vi "new encoder test harness.vi"(5 "input2":bool=TRUE, 6 "Tick Count(Ticks)":u32, 7 "input1":bool=TRUE, 8 "ticks":u32[](array[numeric])=[0, 0], 9 "switch encoders (F)":bool, 10 "rising edge (T)":bool=TRUE, 11 "history in":bool[](array[boolean])=[FALSE, FALSE, FALSE, FALSE, FALSE, FALSE, FALSE, FALSE, FALSE, FALSE, FALSE, FALSE, FALSE, FALSE, FALSE, FALSE, FALSE, FALSE, FALSE, FALSE, FALSE, FALSE, FALSE, FALSE, FALSE, FALSE, FALSE, FALSE, FALSE, FALSE, FALSE, FALSE, FALSE, FALSE, FALSE, FALSE, FALSE, FALSE, FALSE, FALSE, FALSE, FALSE, FALSE, FALSE, FALSE, FALSE, FALSE, FALSE, FALSE, FALSE, FALSE, FALSE, FALSE, FALSE, FALSE, FALSE, FALSE, FALSE, FALSE, FALSE, FALSE, FALSE, FALSE, FALSE, FALSE, FALSE, FALSE, FALSE, FALSE, FALSE, FALSE, FALSE, FALSE, FALSE, FALSE, FALSE, FALSE, FALSE, FALSE, FALSE, FALSE, FALSE, FALSE, FALSE, FALSE, FALSE, FALSE, FALSE, FALSE, FALSE, FALSE, FALSE, FALSE, FALSE, FALSE, FALSE, FALSE, FALSE, FALSE, FALSE]) -> (0 "ticks out":u32[](array[numeric]), 2 "edge detected":bool, 3 "history out":bool[](array[boolean]))   [LabVIEW 2018]
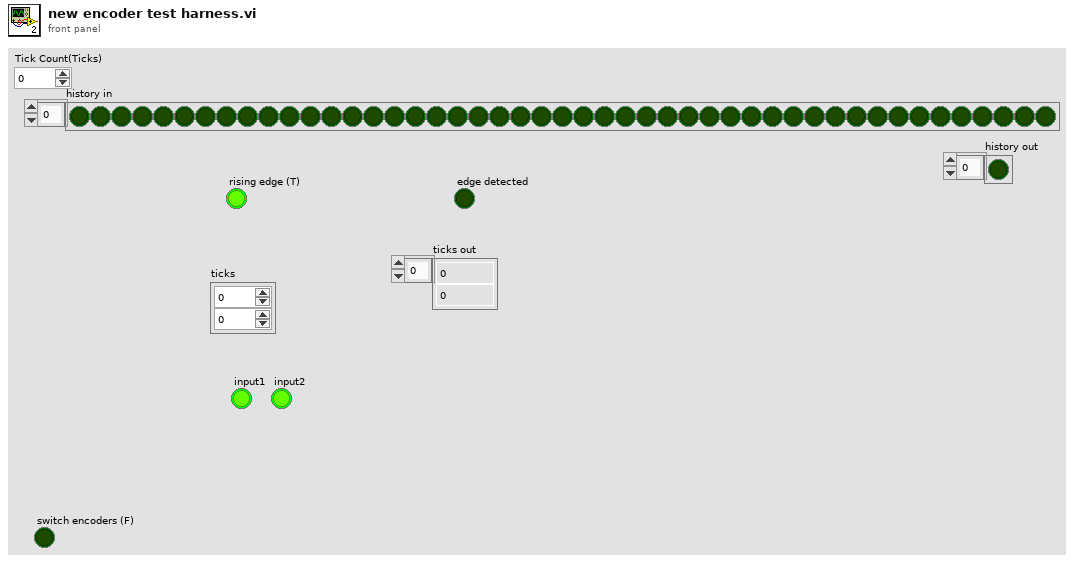
[diagram p1: front panel]
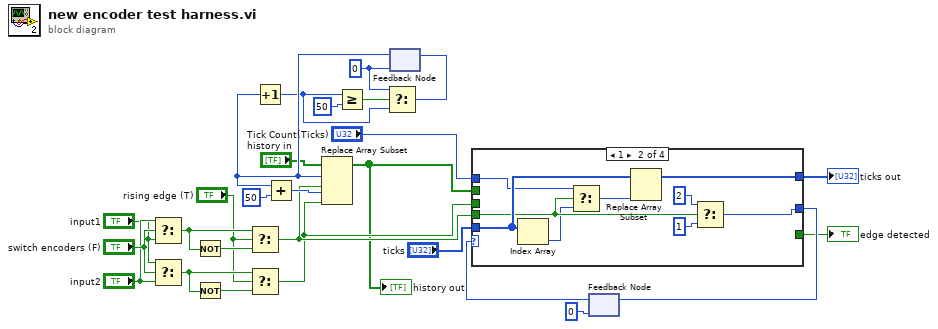
[diagram p0: block diagram]
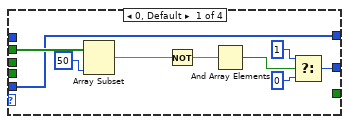
[diagram p2: hidden frame]
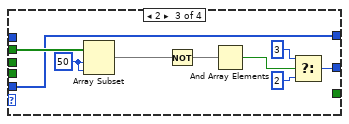
[diagram p3: hidden frame]
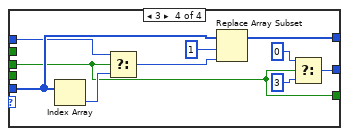
[diagram p4: hidden frame]
diagram:
  w20 = i16 0 ("t")
  n1 = Select(t="input2", s="switch encoders (F)", f="input1") -> (s? t:f=w11:bool)
  n2 = Select(t="input1", s="switch encoders (F)", f="input2") -> (s? t:f=w10:bool)
  n3 = Not(x=w11) -> (.not. x?=w24:bool)
  n4 = Not(x=w10) -> (.not. x?=w23:bool)
  n5 = Select(t=w11, s="rising edge (T)", f=w24) -> (s? t:f=w16:bool)
  n6 = Select(t=w10, s="rising edge (T)", f=w23) -> (s? t:f=w15:bool)
  n7 = feedback #1(w20) -> (w21:i16)
  n8 = Increment(x=w21) -> (x+1=w18:i16)
  n9 = Add(x=w21, y=i16 50) -> (x+y=w27:i16)
  n10 = Replace Array Subset(array="history in", new element #1=w16, index #1=w21, new element #2=w15, index #2=w27) -> (w5:bool[])
  "history out" <- w5
  n11 = Greater Or Equal?(x=w18, y=i16 50 ("x")) -> (x >= y?=w25:bool)
  n12 = Select(t=w20, s=w25, f=w18) -> (s? t:f=w22:i16)
  n13 = feedback-in #1(w22) -> ()
  n14 = feedback #2(u8 0 ("f")) -> (w13:u8)
  n15 = case shown="1" w13 {
    tunnel: w5 -> [w33 _ w51 _]
    tunnel: [w30 w44 w47 w63] -> w14
    tunnel: w16 -> [_ w41 _ _]
    tunnel: w15 -> [_ _ _ w55]
    tunnel: "ticks" -> [w28 w43 w46 w60]
    tunnel: [w28 w42 w46 w61] -> w7
    tunnel: "Tick Count(Ticks)" -> [_ w40 _ w57]
    tunnel: [_ _ _ w55] -> w6
    frame 0, Default {
      n16 = Array Subset(array=w33, length=50) -> (w36:bool[])  [unwired: 1 in]
      n17 = Not(x=w36) -> (.not. x?=w35:bool[])
      n18 = And Array Elements(Boolean array=w35) -> (logical AND=w32:bool)
      n19 = Select(t=u8 1 ("next state"), s=w32, f=u8 0 ("next state")) -> (s? t:f=w30:u8)
    }
    frame 1 {
      n20 = Index Array(array=w43) -> (element=w39:u32)  [unwired: 1 in]
      n21 = Select(t=w40, s=w41, f=w39) -> (s? t:f=w38:u32)
      n22 = Replace Array Subset(array=w43, new element=w38) -> (w42:u32[])  [unwired: 1 in]
      n23 = Select(t=u8 2, s=w41, f=u8 1) -> (s? t:f=w44:u8)
    }
    frame 2 {
      w52 = 50 ("length")
      n24 = Array Subset(array=w51, index=w52, length=w52) -> (w54:bool[])
      n25 = Not(x=w54) -> (.not. x?=w53:bool[])
      n26 = And Array Elements(Boolean array=w53) -> (logical AND=w48:bool)
      n27 = Select(t=u8 3, s=w48, f=u8 2) -> (s? t:f=w47:u8)
    }
    frame 3 {
      n28 = Index Array(array=w60) -> (element=w59:u32)  [unwired: 1 in]
      n29 = Select(t=w57, s=w55, f=w59) -> (s? t:f=w58:u32)
      n30 = Replace Array Subset(array=w60, new element=w58, index=1) -> (w61:u32[])
      n31 = Select(t=u8 0, s=w55, f=u8 3) -> (s? t:f=w63:u8)
    }
  }
  "edge detected" <- w6
  "ticks out" <- w7
  n32 = feedback-in #2(w14) -> ()
